vi "Multiple VIs in a Sub panel.vi"() -> ()   [LabVIEW 2015]
doc: "This example shows how to view VIs in a Subpanel control."
panel:
  in  "?":enum32{"Sine Graph", "Random Data Chart"}(tab)
  in  "Stop":bool
  # "Overview: Demonstrates the use of the Subpanel control to display different VI panels.\nInstructions:"
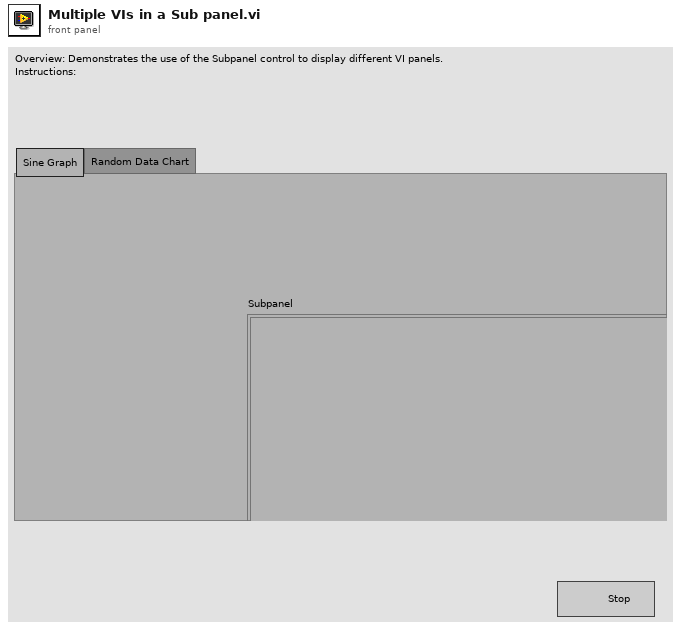
[diagram p1: front panel]
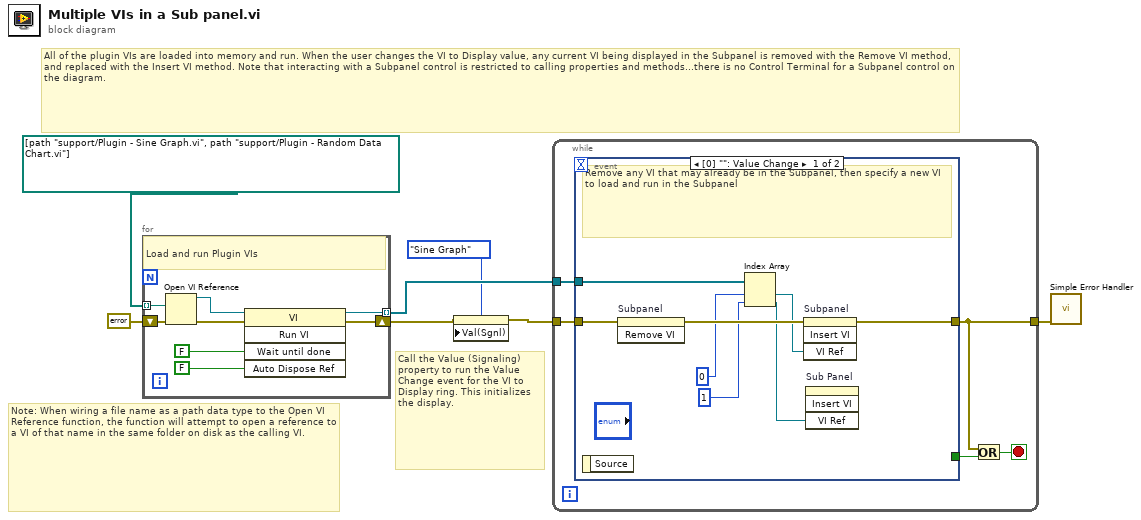
[diagram p0: block diagram]
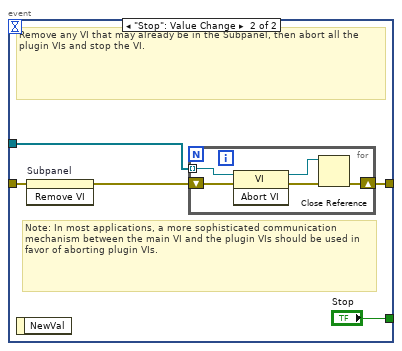
[diagram p2: hidden frame]
diagram:
  # "All of the plugin VIs are loaded into memory and run. When the user changes the VI to Display value, any current VI being displayed in the Subpanel is removed with the Remove VI method, and replaced with the Insert VI method. Note that interacting with a Subpanel control is restricted to calling properties and methods...there is no Control Terminal for a Subpanel control on the diagram."
  # "Note: When wiring a file name as a path data type to the Open VI Reference function, the function will attempt to open a reference to a VI of that name in the same folder on disk as the calling VI."
  # "Call the Value (Signaling) property to run the Value Change event for the VI to Display ring. This initializes the display."
  n1 = for {
    tunnel: path[] [path "support/Plugin - Sine Graph.vi", path "support/Plugin - Random Data Chart.vi"] -> [w11] mode=indexing
    tunnel: [w10] -> w5 mode=indexing
    shift-right: [w8] -> w3
    shift-left: errorcluster {"status"=FALSE, "code"=0, "source"=""} ("error constant") -> [w9]
    # "Load and run Plugin VIs"
    n2 = Open VI Reference(vi path=w11, error in (no error)=w9) -> (vi reference=w12:refnum<vi>, error out=w13:errorcluster)  [unwired: 4 in]
    n3 = invoke class="VI" method="Run VI"(reference=w12, error in=w13, "Wait until done"=FALSE ("Wait Until Done"), "Auto Dispose Ref"=FALSE ("Auto Dispose Reference")) -> (reference out=w10:refnum<vi>, error out=w8:errorcluster)  [unwired: 1 in, 3 out]
  }
  n4 = property class="TabCtl (strict)"(error in=w3, "Val(Sgnl)"=enum32{"Sine Graph", "Random Data Chart"}."Sine Graph" ("Value (Signaling)")) -> (error out=w2:errorcluster)  [unwired: 1 in, 1 out]
  n5 = while {
    tunnel: w2 -> [w16]
    tunnel: [w18] -> w7
    tunnel: w5 -> [w17]
    stop <- w19 stop-if-true
    n6 = event shown="[0] \"\": Value Change" {
      selector: _ -> [_ _]
      dyn-events: _ -> [_ _]
      timeout: _ -> [_ _]
      tunnel: [_ "Stop"] -> w20
      tunnel: [w28 w30] -> w18
      tunnel: w17 -> [w27 w31]
      tunnel: w16 -> [w24 w29]
      event Value Change {
        # "Remove any VI that may already be in the Subpanel, then specify a new VI to load and run in the Subpanel"
        n7 = event-data() -> ()  [unwired: 1 in, 1 out]
        n8 = invoke on="Subpanel" class="SubPnl" method="Remove VI"(error in=w24) -> (error out=w26:errorcluster)  [unwired: 2 in, 2 out]
        n9 = Index Array(array=w27, index #1=0 ("index"), index #2=1 ("index")) -> (element #1=w25:refnum<vi>, element #2=w23:refnum<vi>)
        n10 = invoke on="Subpanel" class="SubPanel" method="Insert VI"(error in=w26, "VI Ref"=w25) -> (error out=w28:errorcluster)  [unwired: 2 in, 3 out]
        n11 = invoke on="Sub Panel" class="SubPnl" method="Insert VI"("VI Ref"=w23) -> ()  [unwired: 3 in, 4 out]
      }
      event "Stop": Value Change {
        # "Note: In most applications, a more sophisticated communication mechanism between the main VI and the plugin VIs should be used in favor of aborting plugin VIs."
        # "Remove any VI that may already be in the Subpanel, then abort all the plugin VIs and stop the VI."
        n12 = event-data() -> ()  [unwired: 1 in, 1 out]
        n13 = invoke on="Subpanel" class="SubPnl" method="Remove VI"(error in=w29) -> (error out=w32:errorcluster)  [unwired: 2 in, 2 out]
        n14 = for {
          shift-right: [w34] -> w30
          shift-left: w32 -> [w38]
          tunnel: w31 -> [w37] mode=indexing
          n15 = invoke class="VI" method="Abort VI"(reference=w37, error in=w38) -> (reference out=w35:refnum<vi>, error out=w36:errorcluster)  [unwired: 1 in, 1 out]
          n16 = Close Reference(reference=w35, error in (no error)=w36) -> (error out=w34:errorcluster)
        }
      }
    }
    n17 = Or(x=w18, y=w20) -> (x .or. y?=w19:bool)
  }
  n18 = call <vilib>:"Simple Error Handler.vi"("error in (no error)"=w7) -> ()  [unwired: 4 in, 5 out]
